vi "create.vi"(7 "manager_daemon in":refnum<class "manager_daemon.lvclass">, 8 "error in (no error)":errorcluster) -> (0 "error out":errorcluster, 3 "manager_daemon out":refnum<class "manager_daemon.lvclass">)   [LabVIEW 2024, in "manager_daemon.lvclass"]
uses:
  manager_daemon.lvclass
  type_defs/msg--cluster.ctl
  type_defs/cmd--enum.ctl
  type_defs/VolumeData--cluster.ctl
  CV_Shared_Library/volume.type--enum.ctl
  type_defs/paths--cluster.ctl
  type_defs/IssueData--clustrer.ctl
  type_defs/sub-map--map.ctl
  type_defs/SubData--cluster.ctl
  CV_Shared_Library/volume.object--cluster.ctl
  TypeDefs/issue.display--cluster.ctl
  manager_daemon.lvclass/manager_daemon.ctl
  CV_Shared_Library/CV_Shared_Library.lvlib
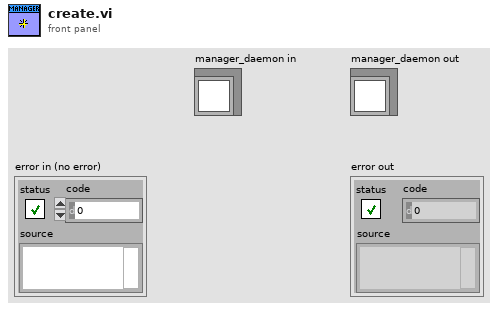
[diagram p1: front panel]
types:
  T1 = map{string, set{cluster{"id":i32, "role":string}}}
  T2 = typedef "CV_Shared_Library.lvlib/volume.object--cluster.ctl" = cluster{"start date":timestamp, "end date":timestamp, "sortable_name":string, "color":u32, "volume type":T3, "issues":T4[]}
  T3 = typedef "CV_Shared_Library.lvlib/volume.type--enum.ctl" = enum16{"Ongoing", "Limited Series", "Annual", "One Shot", "Reprint/Document", "Star Comics", "Epic Comics"}
  T4 = typedef "CV_Shared_Library.lvlib/issue.display--cluster.ctl" = cluster{"cover_date":timestamp, "id":i32, "number":string, "fill":bool}
  T5 = cluster{"filtered data":T2[], "filter dates":cluster{"start":timestamp, "end":timestamp}}
  T6 = typedef "manager_daemon.lvclass/cmd--enum.ctl" = enum16{"init", "run", "load binaries", "build binaries", "save binaries", "create folder map", "display info", "apply filter", "add volume", "update issues", "add issue", "get issues", "get volume", "update volume", "delete volume", "delete issues", "exit"}
  T7 = typedef "manager_daemon.lvclass/sub-map--map.ctl" = map{string, T8}
  T8 = typedef "manager_daemon.lvclass/SubData--cluster.ctl" = cluster{"id":i32, "issues":set{i32}}
  T9 = typedef "manager_daemon.lvclass/IssueData--clustrer.ctl" = cluster{"cover_date":timestamp, "cv_id":string, "name":string, "sortable_name":string, "issue_number":string, "deck":string, "description":string, "id":i32, "store_date":timestamp, "date_last_updated":timestamp, "site_detail_url":string, "cover_url":string, "source_path":path, "character map":map{i32, string}, "concept map":map{i32, string}, "storyArc map":map{i32, string}, "team map":map{i32, string}, "creator map":map{i32, cluster{"name":string, "role":string}}}
  T10 = typedef "manager_daemon.lvclass/paths--cluster.ctl" = cluster{"issue map path":path, "char map path":path, "concept map path":path, "story map path":path, "team map path":path, "volume map path":path, "volumes path":path, "issues path":path, "folder map path":path, "creator map path":path}
  T11 = typedef "manager_daemon.lvclass/VolumeData--cluster.ctl" = cluster{"name":string, "sortable_name":string, "aliases":string[], "description":string, "site_detail_url":string, "count_of_issues":i32, "start_year":i32, "publisher_id":i32, "issue_ids":i32[], "date_last_updated":timestamp, "volume":i32, "cv_id":string, "volume type":T3, "source_path":path}
  T12 = typedef "manager_daemon.lvclass/msg--cluster.ctl" = cluster{"cmd":T6, "data":variant}
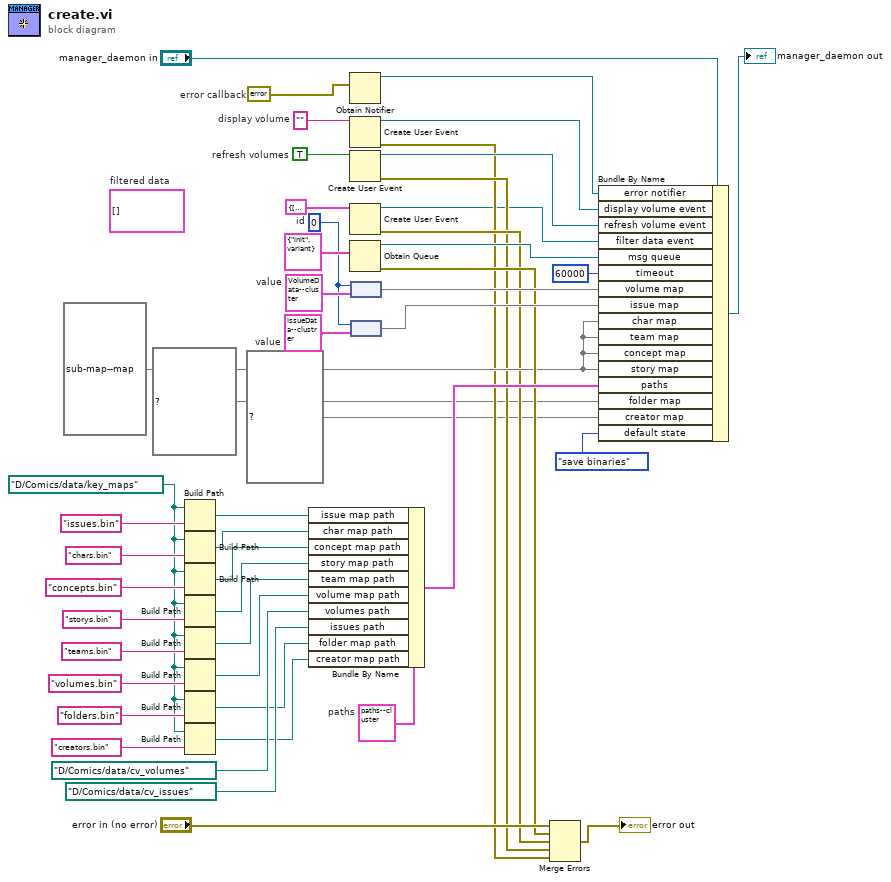
[diagram p0: block diagram]
diagram:
  w11 = errorcluster {"status"=FALSE, "code"=0, "source"=""}  # error callback
  w15 = ""  # display volume
  w19 = TRUE  # refresh volumes
  (unwired) T2[] []  # filtered data
  w20 = T7 {} ("map")
  w21 = 0  # id
  w1 = path "D:/Comics/data/key_maps" ("issue map path")
  w44 = T9 {"cover_date"=timestamp(0 s since 1904-01-01), "cv_id"="", "name"="", "sortable_name"="", "issue_number"="", "deck"="", "description"="", "id"=0, "store_date"=timestamp(0 s since 1904-01-01), "date_last_updated"=timestamp(0 s since 1904-01-01), "site_detail_url"="", "cover_url"="", "source_path"=path "", "character map"={}, "concept map"={}, "storyArc map"={}, "team map"={}, "creator map"={}}  # value
  w40 = T10 {"issue map path"=path "", "char map path"=path "", "concept map path"=path "", "story map path"=path "", "team map path"=path "", "volume map path"=path "", "volumes path"=path "", "issues path"=path "", "folder map path"=path "", "creator map path"=path "D:/Comics/data/key_maps/teams.bin"}  # paths
  w45 = T11 {"name"="", "sortable_name"="", "aliases"=[], "description"="", "site_detail_url"="", "count_of_issues"=0, "start_year"=0, "publisher_id"=0, "issue_ids"=[], "date_last_updated"=timestamp(0 s since 1904-01-01), "volume"=0, "cv_id"="", "volume type"=enum."Ongoing", "source_path"=path ""}  # value
  n1 = Build Path(base path=w1, name or relative path="issues.bin") -> (appended path=w32:path)
  n2 = Build Path(base path=w1, name or relative path="chars.bin") -> (appended path=w31:path)
  n3 = Build Path(base path=w1, name or relative path="concepts.bin") -> (appended path=w30:path)
  n4 = Build Path(base path=w1, name or relative path="storys.bin") -> (appended path=w29:path)
  n5 = Build Path(base path=w1, name or relative path="teams.bin") -> (appended path=w28:path)
  n6 = Build Path(base path=w1, name or relative path="volumes.bin") -> (appended path=w27:path)
  n7 = Build Path(base path=w1, name or relative path="folders.bin") -> (appended path=w6:path)
  n8 = Build Path(base path=w1, name or relative path="creators.bin") -> (appended path=w4:path)
  n9 = Bundle By Name(cluster=w40, "issue map path"=w32, "char map path"=w31, "concept map path"=w30, "story map path"=w29, "team map path"=w28, "volume map path"=w27, "volumes path"=path "D:/Comics/data/cv_volumes" ("issue map path"), "issues path"=path "D:/Comics/data/cv_issues" ("issue map path"), "folder map path"=w6, "creator map path"=w4) -> (w39:T10)
  n10 = Obtain Notifier(notification data type=w11) -> (notifier out=w10:refnum<notifier>)  [unwired: 3 in, 2 out]
  n11 = Create User Event(user event datatype=w15) -> (user event=w14:refnum<user-event>, error out=w13:errorcluster)  [unwired: 1 in]
  n12 = Create User Event(user event datatype=w19) -> (user event=w18:refnum<user-event>, error out=w16:errorcluster)  [unwired: 1 in]
  n13 = Create User Event(user event datatype=T5 {"filtered data"=[], "filter dates"={"start"=timestamp(0 s since 1904-01-01), "end"=timestamp(0 s since 1904-01-01)}} ("filter results")) -> (user event=w8:refnum<user-event>, error out=w17:errorcluster)  [unwired: 1 in]
  n14 = Obtain Queue(element data type=T12 {"cmd"=enum."init", "data"=variant} ("msg")) -> (queue out=w46:refnum<queue>, error out=w22:errorcluster)  [unwired: 4 in, 1 out]
  n15 = node(w21, w45) -> (w42:map{i32, T11})
  n16 = node(w21, w44) -> (w41:map{i32, T9})
  n17 = Merge Errors("error in (no error)", w22, w17, w16, w13) -> (→"error out":errorcluster)
  n18 = Bundle By Name(cluster="manager_daemon in", "error notifier"=w10, "display volume event"=w14, "refresh volume event"=w18, "filter data event"=w8, "msg queue"=w46, "timeout"=60000, "volume map"=w42, "issue map"=w41, "char map"=w20, "team map"=w20, "concept map"=w20, "story map"=w20, "paths"=w39, "folder map"=map{i32, map{string, i32}} {}, "creator map"=T1 {}, "default state"=cmd--enum."save binaries") -> (→"manager_daemon out":refnum<class "manager_daemon.lvclass">)
